vi "ApproachingStep(NoZFeedback).vi"() -> ()   [LabVIEW 2014]
uses:
  <vilib>/Platform/TimedLoop/XDataNode/timing_clust.ctl
  <vilib>/Platform/TimedLoop/XDataNode/nitl_modes.ctl
  <vilib>/Platform/TimedLoop/XDataNode/wakeup.ctl
  <vilib>/rvi/Emulation/niFpgaSctlEmulationGetInTimedLoop.vi
  <vilib>/rvi/Emulation/niFpgaProcessEmulError.vi
  <vilib>/rvi/eio/common/nirviEmuTemplateMethod_errors.vi
  <vilib>/rvi/Emulation/niFpgaGetClockAttributes.vi
  <vilib>/rvi/Emulation/niFpgaEmulationReportErrorSimple.vi
  <vilib>/rvi/Emulation/niFpgaCriticalErrorInLSC.vi
  <vilib>/eio/EIONode/EIONode.xnode
  <vilib>/Platform/TimedLoop/XDataNode/XDataNode.xnode
  <vilib>/Platform/TimedLoop/XDataNode/XDNodeRunTimeDep.lvlib
panel:
  in  "Threshold":sgl=0.0035
  in  "DefaultThreshold?":bool=TRUE
  in  "Count(uSec)":u32=250
  out "ZCalPos":i32
  out "Approached?":bool
  out "PIZRangeExceeded?":bool
  out "ExceedUpperLimit?":bool
  out "RealPIZPos":i16
  out "PresCurr":i16
  in  "stop":bool
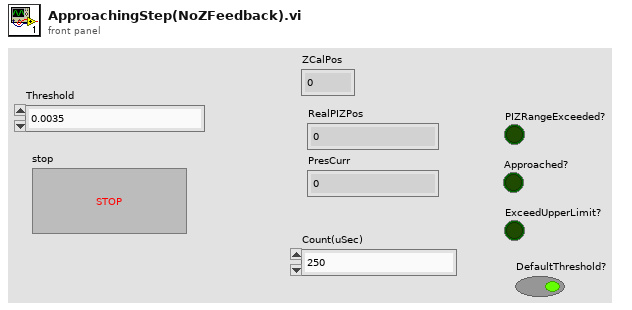
[diagram p1: front panel]
types:
  T1 = typedef "XDNodeRunTimeDep.lvlib/timing_clust.ctl" = cluster{"Expected End [f-1]":u64, "Actual End [f-1]":u64, "Finished Late? [f-1]":bool, "Expected End [i-1]":u64, "Actual End [i-1]":u64, "Finished Late? [i-1]":bool, "Expected Start [i]":u64, "Actual Start [i]":u64, "Expected Start [f]":u64, "Actual Start [f]":u64, "Source Name":string, "Structure Name":string, "Period":i64, "Deadline":i64, "Offset":i64, "Start":i64, "Priority":i32, "Timeout":i32, "Mode":T2, "Wakeup Reason":T3, "Error":errorcluster, "Source Type":string, "Secondary Source Type":string, "Global End Time":u64, "Global Start Time":u64, "Frame Duration":u64, "Iteration Duration":u64, "Assigned CPU":i32, "I/O Scan Engine Mode":u32}
  T2 = typedef "XDNodeRunTimeDep.lvlib/nitl_modes.ctl" = enum32{"No Change", "Process missed periods, maintain original phase", "Discard missed periods, maintain original phase", "Process missed periods, ignore original phase", "Discard missed periods, ignore original phase"}
  T3 = typedef "XDNodeRunTimeDep.lvlib/wakeup.ctl" = enum32{"Normal", "Aborted", "Asynchronous wakeup", "Timing source error", "Timed loop error", "Timeout"}
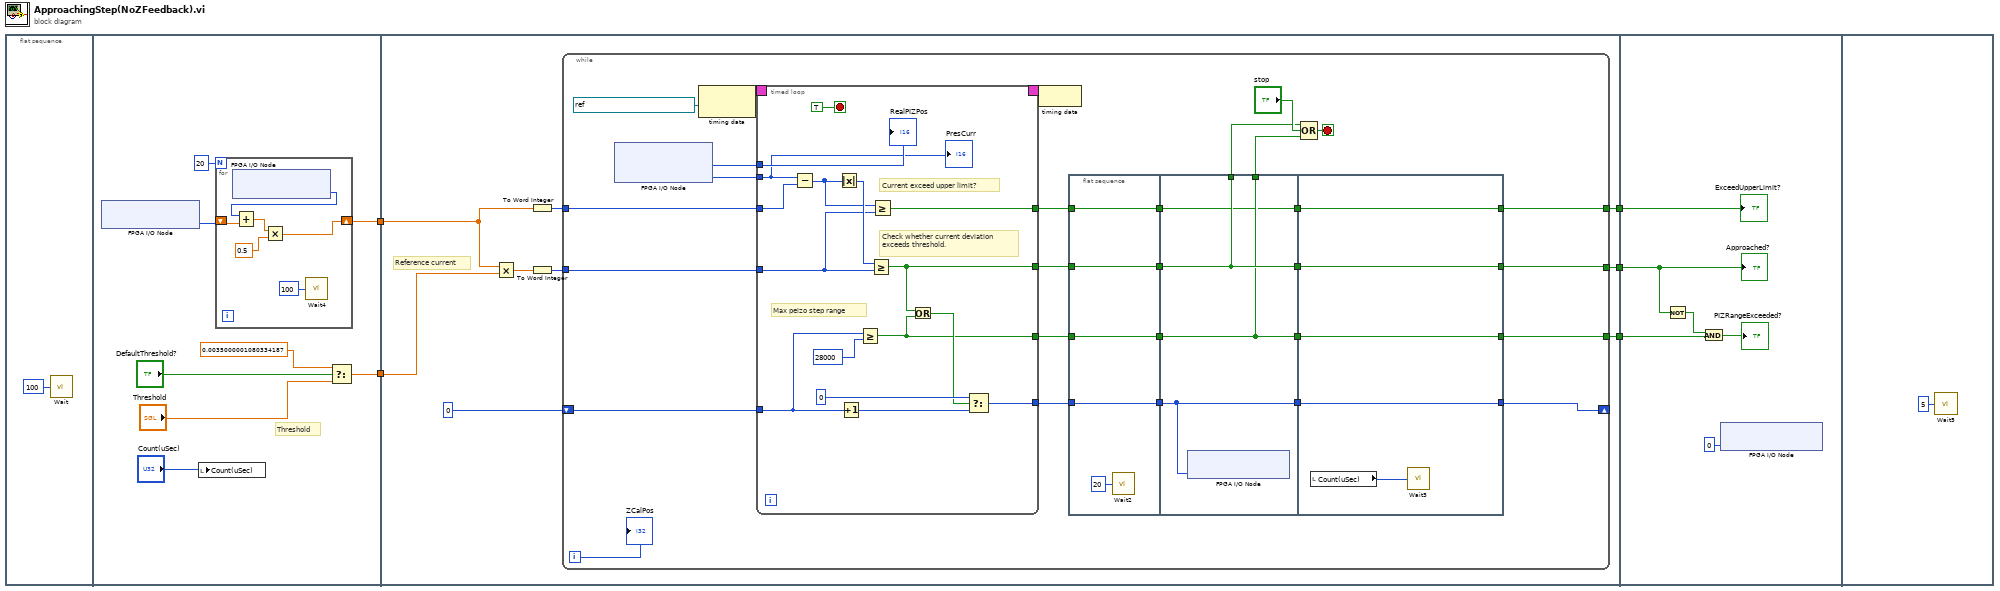
[diagram p0: block diagram]
diagram:
  n1 = flat-sequence {
    tunnel: [w12] -> w2
    tunnel: [w7] -> w1
    tunnel: [w28] -> w5
    tunnel: [w27] -> w4
    tunnel: [w26] -> w3
    tunnel: w2 -> [w23]
    tunnel: w1 -> [w21]
    tunnel: w5 -> [w98]
    tunnel: w4 -> [w100]
    tunnel: w3 -> [w96]
    frame #0 {
      n2 = call "Wait"("Count(uSec)"=u32 100) -> ()  [unwired: 1 out]
    }
    frame #1 {
      # "Threshold"
      n3 = xnode "FPGA I/O Node"() -> ("Connector0/AI1"=w13:i16)  [unwired: 1 in, 1 out]
      n4 = local write "Count(uSec)"("Count(uSec)") -> ()
      n5 = for {
        N: 20 -> [_]
        shift-right: [w16] -> w12
        shift-left: w13 -> [w20]
        n6 = xnode "FPGA I/O Node"() -> ("Connector0/AI1"=w19:i16)  [unwired: 1 in, 1 out]
        n7 = Add(x=w19, y=w20) -> (x+y=w18:sgl)
        n8 = Multiply(x=w18, y=sgl 0.5) -> (x*y=w16:sgl)
        n9 = call "Wait4"("Count(uSec)"=u32 100) -> ()  [unwired: 1 out]
      }
      n10 = Select(t=sgl 0.0035, s="DefaultThreshold?", f="Threshold") -> (s? t:f=w7:sgl)
    }
    frame #2 {
      # "Reference current"
      n11 = Multiply(x=w23, y=w21) -> (x*y=w25:sgl)
      n12 = To Word Integer(number=w23) -> (16bit integer=w22:i16)
      n13 = To Word Integer(number=w25) -> (16bit integer=w24:i16)
      n14 = while {
        tunnel: w24 -> [w50]
        tunnel: w22 -> [w49]
        tunnel: [w34] -> w28
        tunnel: [w33] -> w27
        tunnel: [w35] -> w26
        shift-right: [w31] -> _
        shift-left: i16 0 -> [w51]
        i -> [w30]
        stop <- w52 stop-if-true
        n15 = xnode "FPGA I/O Node"() -> ("Connector0/AI0"=w55:i16, "Connector0/AI1"=w54:i16)  [unwired: 2 in, 2 out]
        n16 = node-c288(refnum<k21> "40 MHz Onboard Clock" ("Source Name")) -> (w58:T1)
        n17 = timed-loop {
          timing: w58 -> [_]
          timing-out: [_] -> w57
          tunnel: w49 -> [w73]
          tunnel: w50 -> [w76]
          tunnel: w55 -> [w87]
          tunnel: w54 -> [w74]
          tunnel: [w78] -> w43
          tunnel: w51 -> [w80]
          tunnel: [w84] -> w47
          tunnel: [w81] -> w45
          tunnel: [w75] -> w36
          stop <- TRUE stop-if-true
          # "Current exceed upper limit?"
          # "Max peizo step range"
          # "Check whether current deviation\nexceeds threshold."
          n18 = Subtract(x=w74, y=w73) -> (x-y=w77:i16)
          n19 = Absolute Value(x=w77) -> (abs(x)=w79:i16)
          n20 = Increment(x=w80) -> (x+1=w86:i16)
          n21 = Greater Or Equal?(x=w80, y=i16 28000) -> (x >= y?=w81:bool)
          n22 = Greater Or Equal?(x=w79, y=w76) -> (x >= y?=w78:bool)
          n23 = Greater Or Equal?(x=w77, y=w76) -> (x >= y?=w75:bool)
          n24 = Or(x=w78, y=w81) -> (x .or. y?=w83:bool)
          n25 = Select(t=i16 0, s=w83, f=w86) -> (s? t:f=w84:i16)
          "RealPIZPos" <- w87
          "PresCurr" <- w74
        }
        n26 = node-c288(w57) -> ()
        n27 = flat-sequence {
          tunnel: [w62] -> w48
          tunnel: w47 -> [w62]
          tunnel: [w61] -> w46
          tunnel: w45 -> [w61]
          tunnel: [w60] -> w44
          tunnel: w43 -> [w60]
          tunnel: [w59] -> w37
          tunnel: w36 -> [w59]
          tunnel: w48 -> [w64]
          tunnel: w46 -> [w66]
          tunnel: w44 -> [w67]
          tunnel: [w67] -> w42
          tunnel: [w66] -> w41
          tunnel: [w67] -> w40
          tunnel: [w66] -> w39
          tunnel: [w65] -> w38
          tunnel: w37 -> [w65]
          tunnel: [w64] -> w32
          tunnel: w40 -> [w71]
          tunnel: w39 -> [w70]
          tunnel: w38 -> [w72]
          tunnel: [w72] -> w35
          tunnel: [w71] -> w34
          tunnel: [w70] -> w33
          tunnel: w32 -> [w69]
          tunnel: [w69] -> w31
          frame #0 {
            n28 = call "Wait2"("Count(uSec)"=u32 20) -> ()  [unwired: 1 out]
          }
          frame #1 {
            n29 = xnode "FPGA I/O Node"("Connector0/AO0"=w64) -> ()  [unwired: 1 in, 1 out]
          }
          frame #2 {
            n30 = local read "Count(uSec)"() -> (w68:u32)
            n31 = call "Wait3"("Count(uSec)"=w68) -> ()  [unwired: 1 out]
          }
        }
        n32 = Compound Arithmetic op=OR(w42, "stop", w41) -> (w52:bool)
        "ZCalPos" <- w30
      }
    }
    frame #3 {
      n33 = Not(x=w98) -> (.not. x?=w97:bool)
      n34 = And(x=w97, y=w100) -> (x .and. y?=→"PIZRangeExceeded?":bool)
      n35 = xnode "FPGA I/O Node"("Connector0/AO0"=i16 0) -> ()  [unwired: 1 in, 1 out]
      "Approached?" <- w98
      "ExceedUpperLimit?" <- w96
    }
    frame #4 {
      n36 = call "Wait5"("Count(mSec)"=u32 5) -> ()  [unwired: 1 out]
    }
  }
